vi "rqcBob Cascade (Low Level Example).vi"() -> ()   [LabVIEW 2019]
panel:
  in  "Raw Bob's key":path
  out "?":T1
  in  "QBER":dbl
  in  "Alices's port":string
  in  "Alices's IP":string
  out "pyton script path":path=path "../python_scripts/cascade_alice.py"
  in  "error in":errorcluster
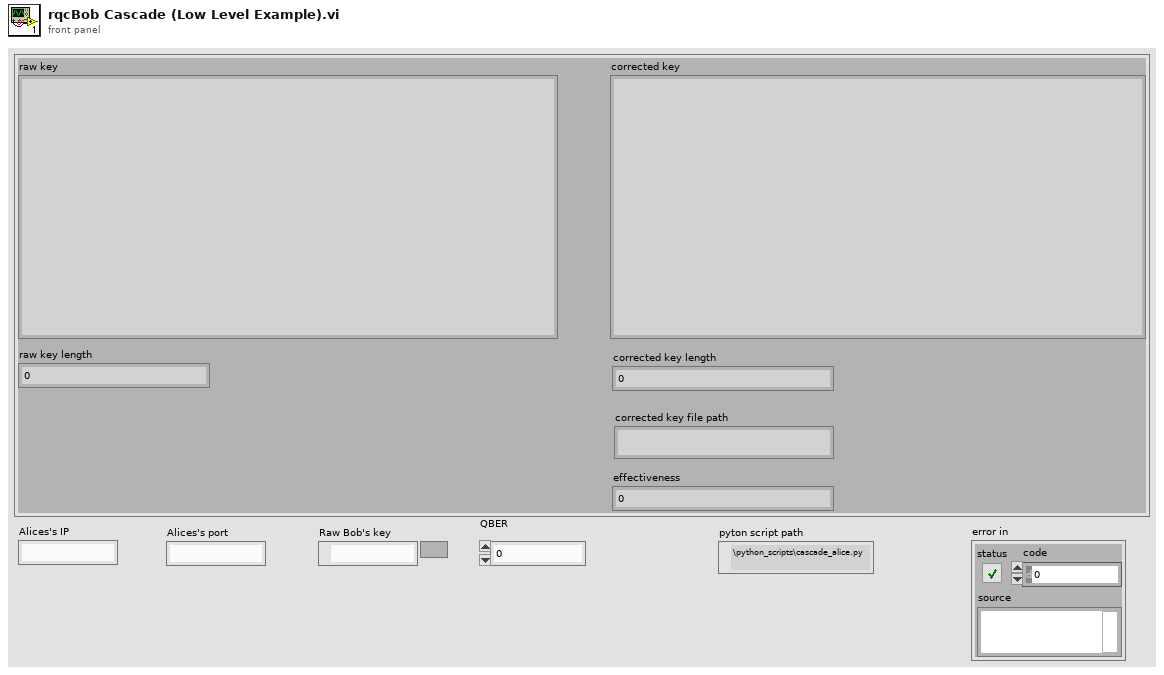
[diagram p1: front panel]
types:
  T1 = cluster{"raw key length":i32, "corrected key":string, "corrected key file path":string, "corrected key length":i32, "effectiveness":dbl, "raw key":string}
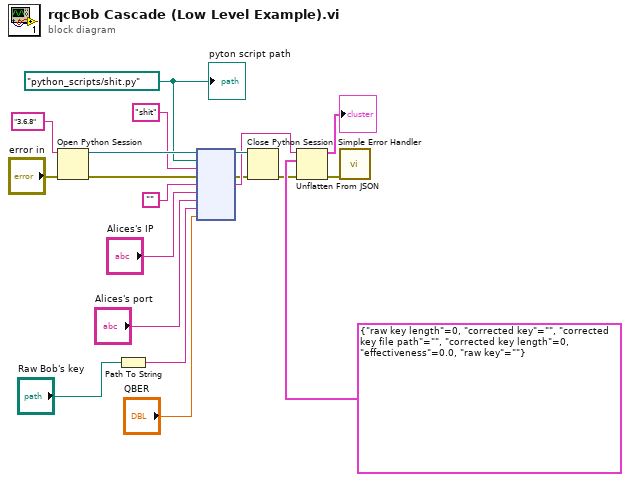
[diagram p0: block diagram]
diagram:
  w13 = path "python_scripts/shit.py" ("module path")
  n1 = Open Python Session(python version="3.6.8" ("Python version"), 3:"error in") -> (session out=w17:refnum<k35>, error out=w16:errorcluster)  [unwired: 1 in]
  n2 = Path To String(path="Raw Bob's key") -> (string=w1:string)
  n3 = node(w17, w13, "shit" ("function name"), w16, "", "Alices's IP", "Alices's port", w1, "QBER") -> (w15:refnum<k35>, w5:errorcluster, w9:string)  [unwired: 4 in, 2 out]
  n4 = Close Python Session(session in=w15, error in=w5) -> (11:w4:errorcluster)
  n5 = Unflatten From JSON(JSON string=w9, type and defaults=T1 {"raw key length"=0, "corrected key"="", "corrected key file path"="", "corrected key length"=0, "effectiveness"=0.0, "raw key"=""}, error in (no error)=w4) -> (value=→"?":T1, error out=w3:errorcluster)  [unwired: 4 in]
  n6 = call <vilib>:"Simple Error Handler.vi"("error in (no error)"=w3) -> ()  [unwired: 4 in, 5 out]
  "pyton script path" <- w13
